vi "Head Co-ordinates 2.vi"(4 "3D Convention":T2(ring), 5 "3D Type and Co-ordinate System":T1(ring), 6 "Sample Rate":dbl format="%.2f", 7 "Array":dbl[][](array[numeric]) format="%.2f") -> (2 "Channel List":string[](array[string]), 3 "3D Output":dbl[][](array[numeric]) format="%.2f")   [LabVIEW 2013]
uses:
  <vilib>/Analysis/baseanly.llb/Real A x B.vi
  <vilib>/Analysis/baseanly.llb/Real Inverse Matrix.vi
  quaternion/quaternion.lvlib
  fick-matrix/fick-matrix.lvlib
  <vilib>/Analysis/NI_AALBase.lvlib
panel:
  # "Copyright Americo A. Migliaccio (c) 2002 All Rights Reserved by Author"
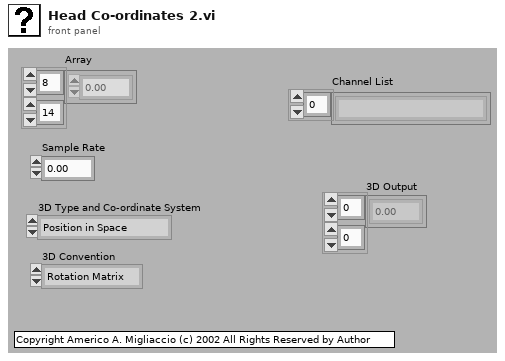
[diagram p1: front panel]
types:
  T1 = enum16{"Position in Space", "Position in Head", "Position in Eye", "Velocity in Space", "Velocity in Head", "Velocity in Eye", "Acceleration in Space", "Acceleration in Head"}
  T2 = enum16{"Rotation Matrix", "Rotation Vectors", "Quaternions", "Fick Angles", "Helmholtz Angles"}
  T3 = typedef "NI_Matrix.lvlib/RealMatrix.ctl" = dbl[][]
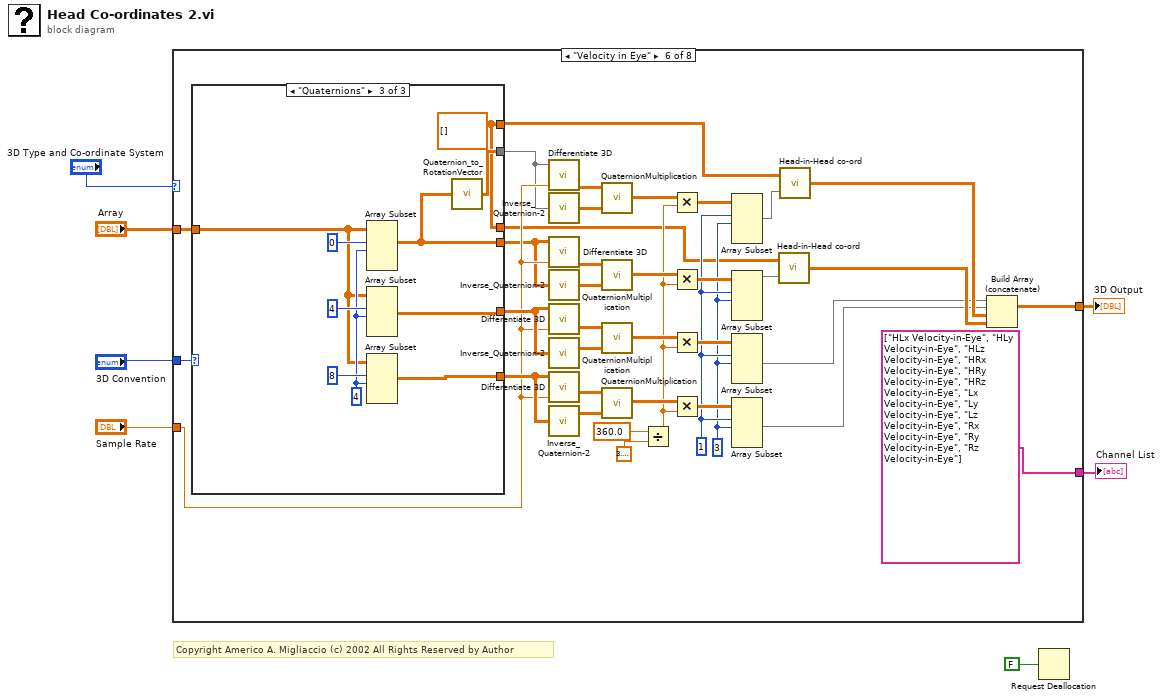
[diagram p0: block diagram]
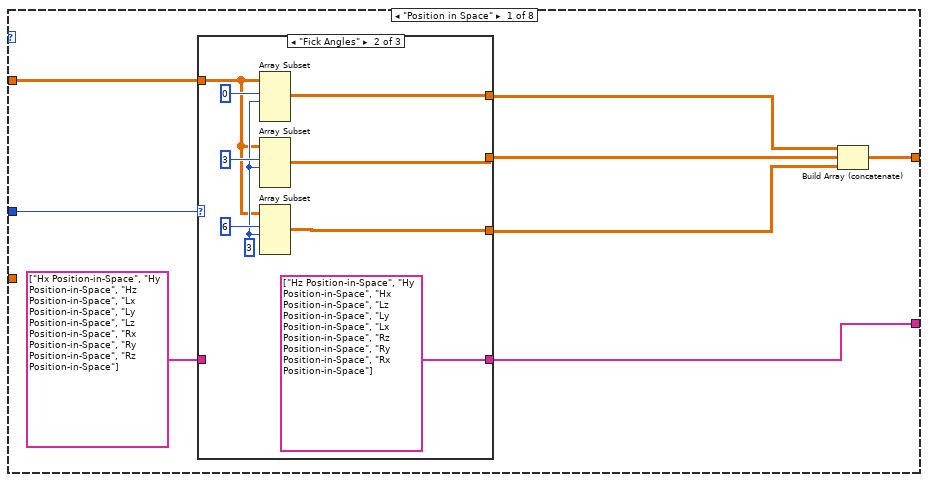
[diagram p2: hidden frame]
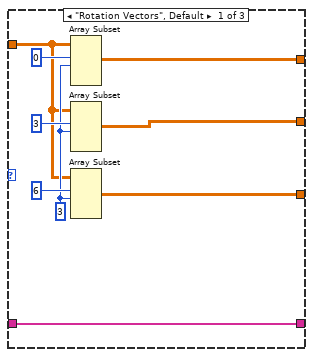
[diagram p3: hidden frame]
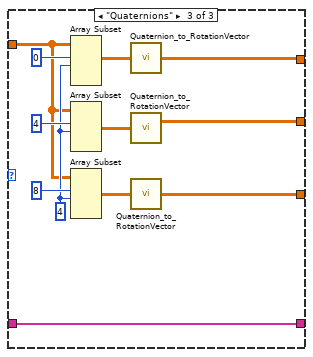
[diagram p4: hidden frame]
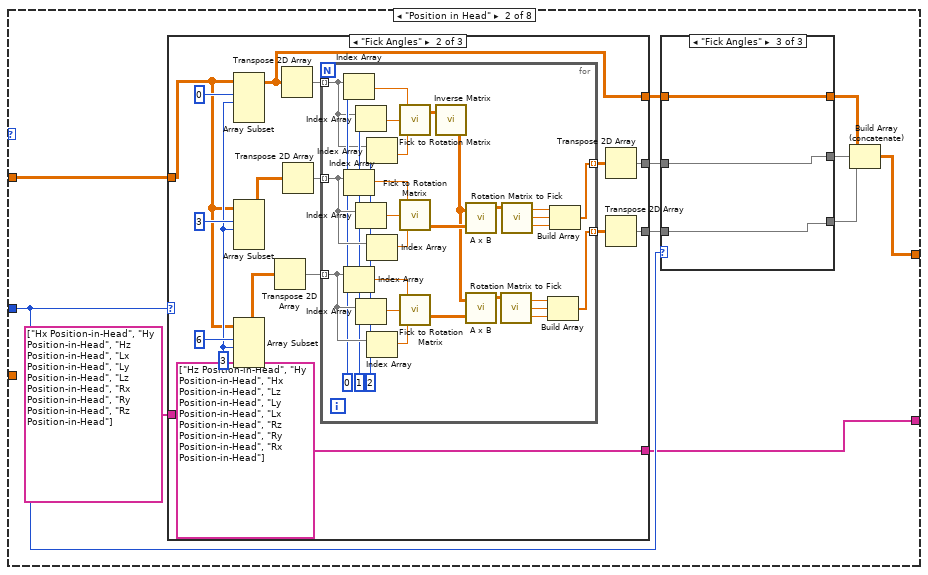
[diagram p5: hidden frame]
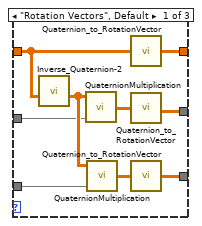
[diagram p6: hidden frame]
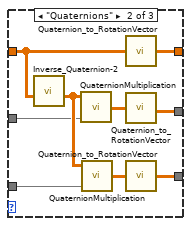
[diagram p7: hidden frame]
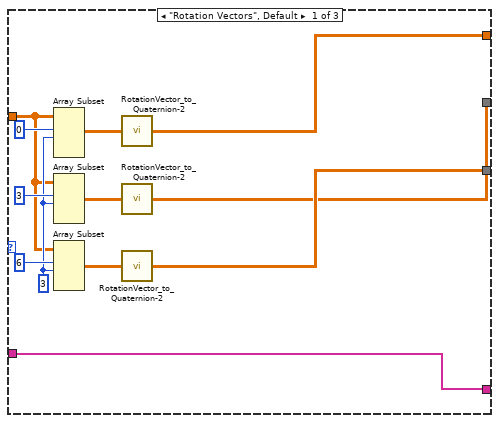
[diagram p8: hidden frame]
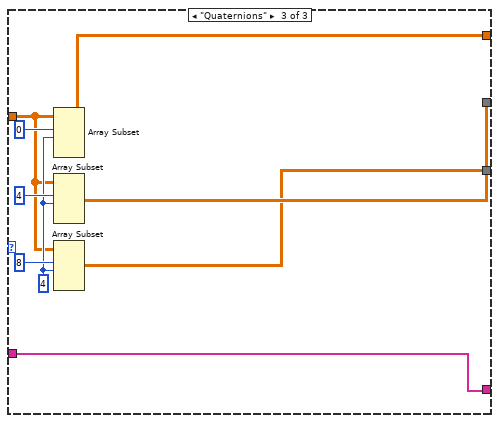
[diagram p9: hidden frame]
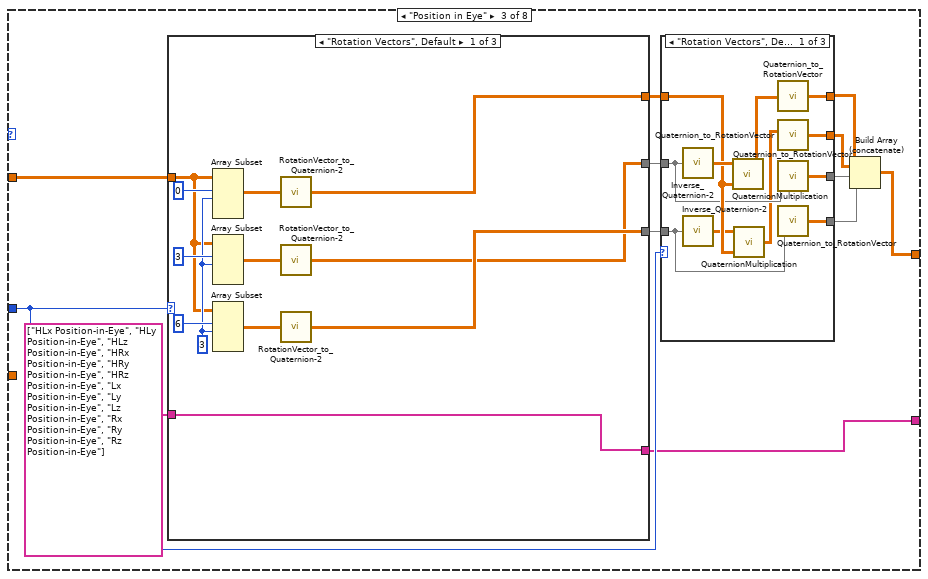
[diagram p10: hidden frame]
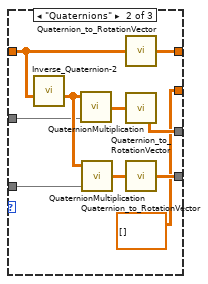
[diagram p11: hidden frame]
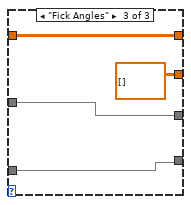
[diagram p12: hidden frame]
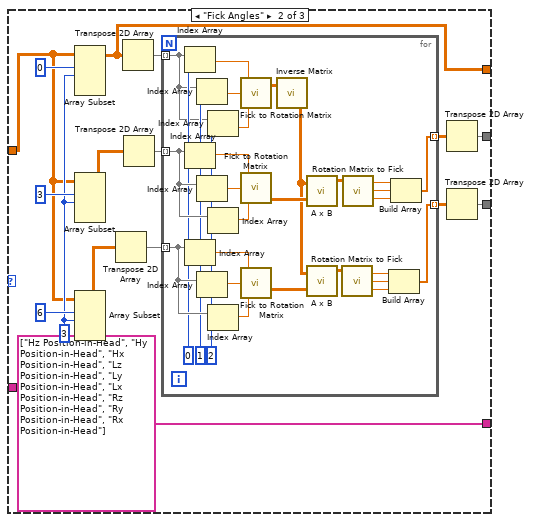
[diagram p13: hidden frame]
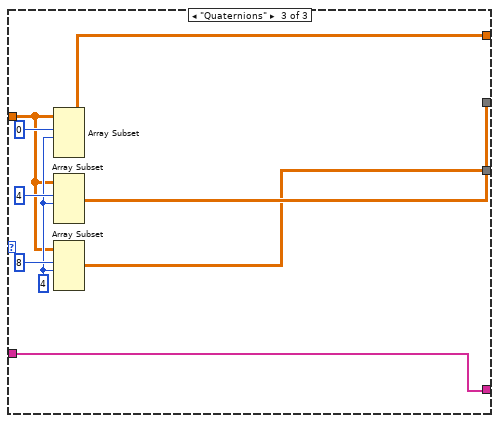
[diagram p14: hidden frame]
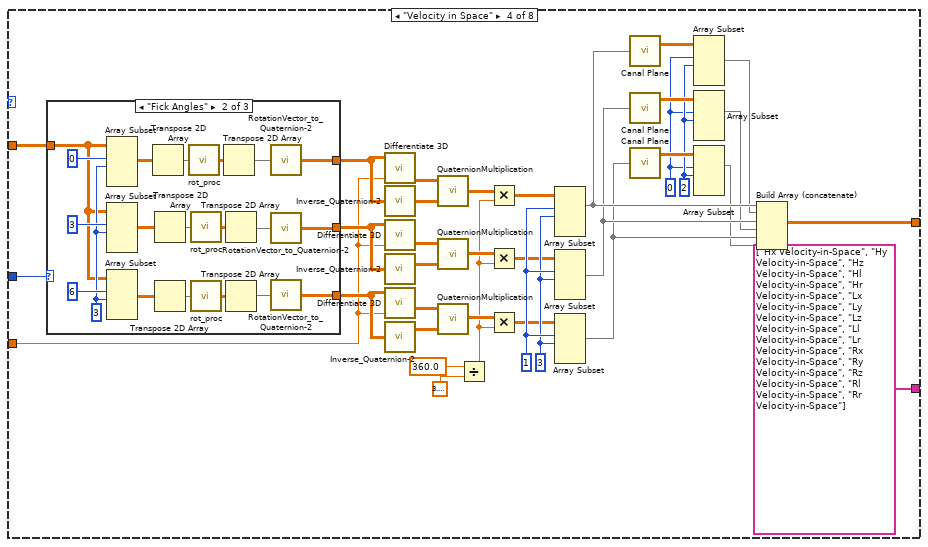
[diagram p15: hidden frame]
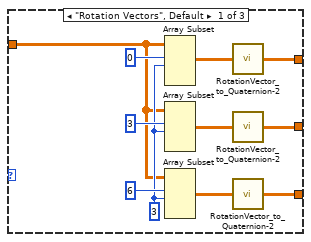
[diagram p16: hidden frame]
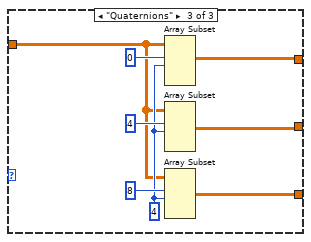
[diagram p17: hidden frame]
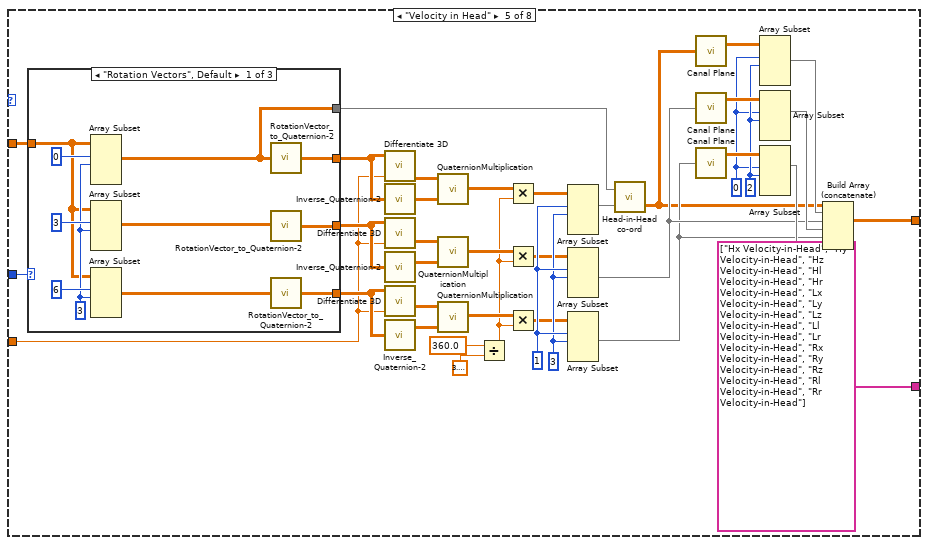
[diagram p18: hidden frame]
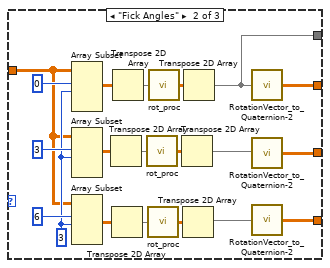
[diagram p19: hidden frame]
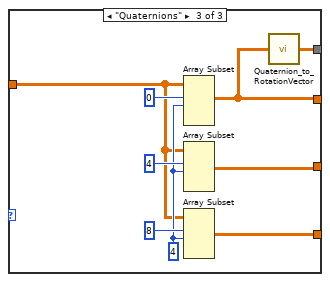
[diagram p20: hidden frame]
diagram:
  # "Copyright Americo A. Migliaccio (c) 2002 All Rights Reserved by Author"
  n1 = case shown="\"Velocity in Eye\"" "3D Type and Co-ordinate System" {
    tunnel: [w10 w50 w150 w263 w327 w420 w484 w498] -> w2
    tunnel: "Array" -> [w15 w48 w148 w282 w359 w437 w496 w510]
    tunnel: "3D Convention" -> [w14 w49 w149 w281 w358 w436 _ _]
    tunnel: "Sample Rate" -> [_ _ _ w264 w338 w408 w488 w502]
    tunnel: [w8 w47 w147 string[] ["Hx Velocity-in-Space", "Hy Velocity-in-Space", "Hz Velocity-in-Space", "Hl Velocity-in-Space", "Hr Velocity-in-Space", "Lx Velocity-in-Space", "Ly Velocity-in-Space", "Lz Velocity-in-Space", "Ll Velocity-in-Space", "Lr Velocity-in-Space", "Rx Velocity-in-Space", "Ry Velocity-in-Space", "Rz Velocity-in-Space", "Rl Velocity-in-Space", "Rr Velocity-in-Space"] ("Channel List") string[] ["Hx Velocity-in-Head", "Hy Velocity-in-Head", "Hz Velocity-in-Head", "Hl Velocity-in-Head", "Hr Velocity-in-Head", "Lx Velocity-in-Head", "Ly Velocity-in-Head", "Lz Velocity-in-Head", "Ll Velocity-in-Head", "Lr Velocity-in-Head", "Rx Velocity-in-Head", "Ry Velocity-in-Head", "Rz Velocity-in-Head", "Rl Velocity-in-Head", "Rr Velocity-in-Head"] ("Channel List") string[] ["HLx Velocity-in-Eye", "HLy Velocity-in-Eye", "HLz Velocity-in-Eye", "HRx Velocity-in-Eye", "HRy Velocity-in-Eye", "HRz Velocity-in-Eye", "Lx Velocity-in-Eye", "Ly Velocity-in-Eye", "Lz Velocity-in-Eye", "Rx Velocity-in-Eye", "Ry Velocity-in-Eye", "Rz Velocity-in-Eye"] ("Channel List") string[] ["Hx Acceleration-in-Space", "Hy Acceleration-in-Space", "Hz Acceleration-in-Space", "Hl Acceleration-in-Space", "Hr Acceleration-in-Space", "Lx Acceleration-in-Space", "Ly Acceleration-in-Space", "Lz Acceleration-in-Space", "Ll Acceleration-in-Space", "Lr Acceleration-in-Space", "Rx Acceleration-in-Space", "Ry Acceleration-in-Space", "Rz Acceleration-in-Space", "Rl Acceleration-in-Space", "Rr Acceleration-in-Space"] ("Channel List") string[] ["Hx Acceleration-in-Head", "Hy Acceleration-in-Head", "Hz Acceleration-in-Head", "Hl Acceleration-in-Head", "Hr Acceleration-in-Head", "Lx Acceleration-in-Head", "Ly Acceleration-in-Head", "Lz Acceleration-in-Head", "Ll Acceleration-in-Head", "Lr Acceleration-in-Head", "Rx Acceleration-in-Head", "Ry Acceleration-in-Head", "Rz Acceleration-in-Head", "Rl Acceleration-in-Head", "Rr Acceleration-in-Head"] ("Channel List")] -> w3
    frame "Position in Space" {
      n2 = case shown="\"Fick Angles\"" w14 {
        tunnel: w15 -> [w20 w29 w41]
        tunnel: [w19 w26 w35] -> w13
        tunnel: [w18 w27 w36] -> w11
        tunnel: [w17 w28 w37] -> w12
        tunnel: string[] ["Hx Position-in-Space", "Hy Position-in-Space", "Hz Position-in-Space", "Lx Position-in-Space", "Ly Position-in-Space", "Lz Position-in-Space", "Rx Position-in-Space", "Ry Position-in-Space", "Rz Position-in-Space"] ("Channel List") -> [w16 _ w34]
        tunnel: [w16 string[] ["Hz Position-in-Space", "Hy Position-in-Space", "Hx Position-in-Space", "Lz Position-in-Space", "Ly Position-in-Space", "Lx Position-in-Space", "Rz Position-in-Space", "Ry Position-in-Space", "Rx Position-in-Space"] ("Channel List") w34] -> w8
        frame "Rotation Vectors", Default {
          w21 = 3 ("Array Length")
          n3 = Array Subset(array=w20, index (row)=0 ("Array Index"), length (row)=w21) -> (w19:dbl[][])  [unwired: 2 in]
          n4 = Array Subset(array=w20, index (row)=3 ("Array Index"), length (row)=w21) -> (w18:dbl[][])  [unwired: 2 in]
          n5 = Array Subset(array=w20, index (row)=6 ("Array Index"), length (row)=w21) -> (w17:dbl[][])  [unwired: 2 in]
        }
        frame "Fick Angles" {
          w30 = 3 ("Array Length")
          n6 = Array Subset(array=w29, index (row)=0 ("Array Index"), length (row)=w30) -> (w26:dbl[][])  [unwired: 2 in]
          n7 = Array Subset(array=w29, index (row)=3 ("Array Index"), length (row)=w30) -> (w27:dbl[][])  [unwired: 2 in]
          n8 = Array Subset(array=w29, index (row)=6 ("Array Index"), length (row)=w30) -> (w28:dbl[][])  [unwired: 2 in]
        }
        frame "Quaternions" {
          w42 = 4 ("Array Length")
          n9 = Array Subset(array=w41, index (row)=0 ("Array Index"), length (row)=w42) -> (w40:dbl[][])  [unwired: 2 in]
          n10 = Array Subset(array=w41, index (row)=4 ("Array Index"), length (row)=w42) -> (w39:dbl[][])  [unwired: 2 in]
          n11 = Array Subset(array=w41, index (row)=8 ("Array Index"), length (row)=w42) -> (w38:dbl[][])  [unwired: 2 in]
          n12 = call "Quaternion_to_RotationVector.vi"("quaternions"=w40) -> ("rotation vectors"=w35:dbl[][])  [unwired: 4 in]
          n13 = call "Quaternion_to_RotationVector.vi"("quaternions"=w39) -> ("rotation vectors"=w36:dbl[][])  [unwired: 4 in]
          n14 = call "Quaternion_to_RotationVector.vi"("quaternions"=w38) -> ("rotation vectors"=w37:dbl[][])  [unwired: 4 in]
        }
      }
      n15 = Build Array (concatenate)(w13, w11, w12) -> (w10:dbl[][])
    }
    frame "Position in Head" {
      n16 = case shown="\"Fick Angles\"" w49 {
        tunnel: w48 -> [w85 w101 w139]
        tunnel: [w79 w91 w138] -> w56
        tunnel: [w80 w93 w137] -> w55
        tunnel: [w81 w92 w136] -> w54
        tunnel: [w78 string[] ["Hz Position-in-Head", "Hy Position-in-Head", "Hx Position-in-Head", "Lz Position-in-Head", "Ly Position-in-Head", "Lx Position-in-Head", "Rz Position-in-Head", "Ry Position-in-Head", "Rx Position-in-Head"] ("Channel List") w135] -> w47
        tunnel: string[] ["Hx Position-in-Head", "Hy Position-in-Head", "Hz Position-in-Head", "Lx Position-in-Head", "Ly Position-in-Head", "Lz Position-in-Head", "Rx Position-in-Head", "Ry Position-in-Head", "Rz Position-in-Head"] ("Channel List") -> [w78 _ w135]
        frame "Rotation Vectors", Default {
          w86 = 3 ("Array Length")
          n17 = Array Subset(array=w85, index (row)=0 ("Array Index"), length (row)=w86) -> (w84:dbl[][])  [unwired: 2 in]
          n18 = Array Subset(array=w85, index (row)=3 ("Array Index"), length (row)=w86) -> (w83:dbl[][])  [unwired: 2 in]
          n19 = Array Subset(array=w85, index (row)=6 ("Array Index"), length (row)=w86) -> (w82:dbl[][])  [unwired: 2 in]
          n20 = call "RotationVector_to_Quaternion-2.vi"("rotation vectors"=w84) -> ("quaternions"=w79:dbl[][])  [unwired: 4 in]
          n21 = call "RotationVector_to_Quaternion-2.vi"("rotation vectors"=w83) -> ("quaternions"=w80:dbl[][])  [unwired: 4 in]
          n22 = call "RotationVector_to_Quaternion-2.vi"("rotation vectors"=w82) -> ("quaternions"=w81:dbl[][])  [unwired: 4 in]
        }
        frame "Fick Angles" {
          w102 = 3 ("Array Length")
          n23 = Array Subset(array=w101, index (row)=0 ("Array Index"), length (row)=w102) -> (w91:dbl[][])  [unwired: 2 in]
          n24 = Array Subset(array=w101, index (row)=3 ("Array Index"), length (row)=w102) -> (w100:dbl[][])  [unwired: 2 in]
          n25 = Array Subset(array=w101, index (row)=6 ("Array Index"), length (row)=w102) -> (w99:dbl[][])  [unwired: 2 in]
          n26 = Transpose 2D Array(2D array=w99) -> (transposed array=w98:dbl[][])
          n27 = Transpose 2D Array(2D array=w91) -> (transposed array=w96:dbl[][])
          n28 = Transpose 2D Array(2D array=w100) -> (transposed array=w97:dbl[][])
          n29 = for {
            tunnel: w96 -> [w110] mode=indexing
            tunnel: w97 -> [w134] mode=indexing
            tunnel: w98 -> [w133] mode=indexing
            tunnel: [w116] -> w95 mode=indexing
            tunnel: [w114] -> w94 mode=indexing
            w130 = 2 ("Array Index")
            w131 = 1 ("Array Index")
            w132 = 0 ("Array Index")
            n30 = Index Array(array=w110, index=w132) -> (element=w113:dbl)
            n31 = Index Array(array=w134, index=w132) -> (element=w127:dbl)
            n32 = Index Array(array=w133, index=w132) -> (element=w124:dbl)
            n33 = Index Array(array=w110, index=w131) -> (element=w112:dbl)
            n34 = Index Array(array=w134, index=w131) -> (element=w128:dbl)
            n35 = Index Array(array=w133, index=w131) -> (element=w126:dbl)
            n36 = Index Array(array=w110, index=w130) -> (element=w111:dbl)
            n37 = Index Array(array=w134, index=w130) -> (element=w129:dbl)
            n38 = Index Array(array=w133, index=w130) -> (element=w125:dbl)
            n39 = call "Fick to Rotation Matrix.vi"("T"=w111, "V"=w112, "H"=w113) -> ("Rotation Matrix"=w123:dbl[][])
            n40 = call "Fick to Rotation Matrix.vi"("T"=w129, "V"=w128, "H"=w127) -> ("Rotation Matrix"=w122:dbl[][])
            n41 = call "Fick to Rotation Matrix.vi"("T"=w125, "V"=w126, "H"=w124) -> ("Rotation Matrix"=w120:dbl[][])
            n42 = call-poly <vilib>:"Inverse Matrix.vi"("Input Matrix"=w123) -> ("Inverse Matrix"=w121:T3)  [unwired: 1 in, 1 out]
            n43 = call-poly <vilib>:"A x B.vi"("B"=w122, "A"=w121) -> ("A x B"=w119:T3)  [unwired: 1 out]
            n44 = call-poly <vilib>:"A x B.vi"("B"=w120, "A"=w121) -> ("A x B"=w118:T3)  [unwired: 1 out]
            n45 = call "Rotation Matrix to Fick.vi"("A"=w118) -> ("T"=w106:dbl, "V"=w115:dbl, "H"=w107:dbl)  [unwired: 2 in]
            n46 = call "Rotation Matrix to Fick.vi"("A"=w119) -> ("T"=w109:dbl, "V"=w117:dbl, "H"=w108:dbl)  [unwired: 2 in]
            n47 = Build Array(w107, w115, w106) -> (w114:dbl[])
            n48 = Build Array(w108, w117, w109) -> (w116:dbl[])
          }
          n49 = Transpose 2D Array(2D array=w95) -> (transposed array=w93:dbl[][])
          n50 = Transpose 2D Array(2D array=w94) -> (transposed array=w92:dbl[][])
        }
        frame "Quaternions" {
          w140 = 4 ("Array Length")
          n51 = Array Subset(array=w139, index (row)=0 ("Array Index"), length (row)=w140) -> (w138:dbl[][])  [unwired: 2 in]
          n52 = Array Subset(array=w139, index (row)=4 ("Array Index"), length (row)=w140) -> (w137:dbl[][])  [unwired: 2 in]
          n53 = Array Subset(array=w139, index (row)=8 ("Array Index"), length (row)=w140) -> (w136:dbl[][])  [unwired: 2 in]
        }
      }
      n54 = case shown="\"Fick Angles\"" w49 {
        tunnel: w56 -> [w62 w71 w75]
        tunnel: w55 -> [w61 w70 w76]
        tunnel: w54 -> [w60 w69 w77]
        tunnel: [w59 w68 w76] -> w53
        tunnel: [w58 w67 w75] -> w52
        tunnel: [w57 w66 w77] -> w51
        frame "Rotation Vectors", Default {
          n55 = call "Inverse_Quaternion-2.vi"("quaternions"=w62) -> ("inverse quaternions"=w64:dbl[][])  [unwired: 4 in]
          n56 = call "QuaternionMultiplication.vi"("quaternions B"=w61, "quaternions A"=w64) -> ("quaternions A x B"=w63:dbl[][])  [unwired: 3 in]
          n57 = call "QuaternionMultiplication.vi"("quaternions B"=w60, "quaternions A"=w64) -> ("quaternions A x B"=w65:dbl[][])  [unwired: 3 in]
          n58 = call "Quaternion_to_RotationVector.vi"("quaternions"=w62) -> ("rotation vectors"=w58:dbl[][])  [unwired: 4 in]
          n59 = call "Quaternion_to_RotationVector.vi"("quaternions"=w63) -> ("rotation vectors"=w59:dbl[][])  [unwired: 4 in]
          n60 = call "Quaternion_to_RotationVector.vi"("quaternions"=w65) -> ("rotation vectors"=w57:dbl[][])  [unwired: 4 in]
        }
        frame "Quaternions" {
          n61 = call "Inverse_Quaternion-2.vi"("quaternions"=w71) -> ("inverse quaternions"=w73:dbl[][])  [unwired: 4 in]
          n62 = call "QuaternionMultiplication.vi"("quaternions B"=w70, "quaternions A"=w73) -> ("quaternions A x B"=w72:dbl[][])  [unwired: 3 in]
          n63 = call "QuaternionMultiplication.vi"("quaternions B"=w69, "quaternions A"=w73) -> ("quaternions A x B"=w74:dbl[][])  [unwired: 3 in]
          n64 = call "Quaternion_to_RotationVector.vi"("quaternions"=w71) -> ("rotation vectors"=w67:dbl[][])  [unwired: 4 in]
          n65 = call "Quaternion_to_RotationVector.vi"("quaternions"=w72) -> ("rotation vectors"=w68:dbl[][])  [unwired: 4 in]
          n66 = call "Quaternion_to_RotationVector.vi"("quaternions"=w74) -> ("rotation vectors"=w66:dbl[][])  [unwired: 4 in]
        }
        frame "Fick Angles" {
        }
      }
      n67 = Build Array (concatenate)(w52, w53, w51) -> (w50:dbl[][])
    }
    frame "Position in Eye" {
      n68 = case shown="\"Rotation Vectors\", Default" w149 {
        tunnel: w148 -> [w188 w204 w242]
        tunnel: [w182 w194 w241] -> w155
        tunnel: [w183 w196 w240] -> w154
        tunnel: [w184 w195 w239] -> w153
        tunnel: [w181 string[] ["Hz Position-in-Head", "Hy Position-in-Head", "Hx Position-in-Head", "Lz Position-in-Head", "Ly Position-in-Head", "Lx Position-in-Head", "Rz Position-in-Head", "Ry Position-in-Head", "Rx Position-in-Head"] ("Channel List") w238] -> w147
        tunnel: string[] ["HLx Position-in-Eye", "HLy Position-in-Eye", "HLz Position-in-Eye", "HRx Position-in-Eye", "HRy Position-in-Eye", "HRz Position-in-Eye", "Lx Position-in-Eye", "Ly Position-in-Eye", "Lz Position-in-Eye", "Rx Position-in-Eye", "Ry Position-in-Eye", "Rz Position-in-Eye"] ("Channel List") -> [w181 _ w238]
        frame "Rotation Vectors", Default {
          w189 = 3 ("Array Length")
          n69 = Array Subset(array=w188, index (row)=0 ("Array Index"), length (row)=w189) -> (w187:dbl[][])  [unwired: 2 in]
          n70 = Array Subset(array=w188, index (row)=3 ("Array Index"), length (row)=w189) -> (w186:dbl[][])  [unwired: 2 in]
          n71 = Array Subset(array=w188, index (row)=6 ("Array Index"), length (row)=w189) -> (w185:dbl[][])  [unwired: 2 in]
          n72 = call "RotationVector_to_Quaternion-2.vi"("rotation vectors"=w187) -> ("quaternions"=w182:dbl[][])  [unwired: 4 in]
          n73 = call "RotationVector_to_Quaternion-2.vi"("rotation vectors"=w186) -> ("quaternions"=w183:dbl[][])  [unwired: 4 in]
          n74 = call "RotationVector_to_Quaternion-2.vi"("rotation vectors"=w185) -> ("quaternions"=w184:dbl[][])  [unwired: 4 in]
        }
        frame "Fick Angles" {
          w205 = 3 ("Array Length")
          n75 = Array Subset(array=w204, index (row)=0 ("Array Index"), length (row)=w205) -> (w194:dbl[][])  [unwired: 2 in]
          n76 = Array Subset(array=w204, index (row)=3 ("Array Index"), length (row)=w205) -> (w203:dbl[][])  [unwired: 2 in]
          n77 = Array Subset(array=w204, index (row)=6 ("Array Index"), length (row)=w205) -> (w202:dbl[][])  [unwired: 2 in]
          n78 = Transpose 2D Array(2D array=w202) -> (transposed array=w201:dbl[][])
          n79 = Transpose 2D Array(2D array=w194) -> (transposed array=w199:dbl[][])
          n80 = Transpose 2D Array(2D array=w203) -> (transposed array=w200:dbl[][])
          n81 = for {
            tunnel: w199 -> [w213] mode=indexing
            tunnel: w200 -> [w237] mode=indexing
            tunnel: w201 -> [w236] mode=indexing
            tunnel: [w219] -> w198 mode=indexing
            tunnel: [w217] -> w197 mode=indexing
            w233 = 2 ("Array Index")
            w234 = 1 ("Array Index")
            w235 = 0 ("Array Index")
            n82 = Index Array(array=w213, index=w235) -> (element=w216:dbl)
            n83 = Index Array(array=w237, index=w235) -> (element=w230:dbl)
            n84 = Index Array(array=w236, index=w235) -> (element=w227:dbl)
            n85 = Index Array(array=w213, index=w234) -> (element=w215:dbl)
            n86 = Index Array(array=w237, index=w234) -> (element=w231:dbl)
            n87 = Index Array(array=w236, index=w234) -> (element=w229:dbl)
            n88 = Index Array(array=w213, index=w233) -> (element=w214:dbl)
            n89 = Index Array(array=w237, index=w233) -> (element=w232:dbl)
            n90 = Index Array(array=w236, index=w233) -> (element=w228:dbl)
            n91 = call "Fick to Rotation Matrix.vi"("T"=w214, "V"=w215, "H"=w216) -> ("Rotation Matrix"=w226:dbl[][])
            n92 = call "Fick to Rotation Matrix.vi"("T"=w232, "V"=w231, "H"=w230) -> ("Rotation Matrix"=w225:dbl[][])
            n93 = call "Fick to Rotation Matrix.vi"("T"=w228, "V"=w229, "H"=w227) -> ("Rotation Matrix"=w223:dbl[][])
            n94 = call-poly <vilib>:"Inverse Matrix.vi"("Input Matrix"=w226) -> ("Inverse Matrix"=w224:T3)  [unwired: 1 in, 1 out]
            n95 = call-poly <vilib>:"A x B.vi"("B"=w225, "A"=w224) -> ("A x B"=w222:T3)  [unwired: 1 out]
            n96 = call-poly <vilib>:"A x B.vi"("B"=w223, "A"=w224) -> ("A x B"=w221:T3)  [unwired: 1 out]
            n97 = call "Rotation Matrix to Fick.vi"("A"=w221) -> ("T"=w209:dbl, "V"=w218:dbl, "H"=w210:dbl)  [unwired: 2 in]
            n98 = call "Rotation Matrix to Fick.vi"("A"=w222) -> ("T"=w212:dbl, "V"=w220:dbl, "H"=w211:dbl)  [unwired: 2 in]
            n99 = Build Array(w210, w218, w209) -> (w217:dbl[])
            n100 = Build Array(w211, w220, w212) -> (w219:dbl[])
          }
          n101 = Transpose 2D Array(2D array=w198) -> (transposed array=w196:dbl[][])
          n102 = Transpose 2D Array(2D array=w197) -> (transposed array=w195:dbl[][])
        }
        frame "Quaternions" {
          w243 = 4 ("Array Length")
          n103 = Array Subset(array=w242, index (row)=0 ("Array Index"), length (row)=w243) -> (w241:dbl[][])  [unwired: 2 in]
          n104 = Array Subset(array=w242, index (row)=4 ("Array Index"), length (row)=w243) -> (w240:dbl[][])  [unwired: 2 in]
          n105 = Array Subset(array=w242, index (row)=8 ("Array Index"), length (row)=w243) -> (w239:dbl[][])  [unwired: 2 in]
        }
      }
      n106 = case shown="\"Rotation Vectors\", Default" w149 {
        tunnel: w155 -> [w161 w173 w178]
        tunnel: w154 -> [w158 w172 w179]
        tunnel: w153 -> [w159 w171 w180]
        tunnel: [w166 w170 w179] -> w152
        tunnel: [w165 w169 w178] -> w145
        tunnel: [w164 w168 w180] -> w151
        tunnel: [w163 dbl[][] [] ("rotation vectors") dbl[][] [] ("rotation vectors")] -> w144
        frame "Rotation Vectors", Default {
          n107 = call "Inverse_Quaternion-2.vi"("quaternions"=w158) -> ("inverse quaternions"=w162:dbl[][])  [unwired: 4 in]
          n108 = call "Inverse_Quaternion-2.vi"("quaternions"=w159) -> ("inverse quaternions"=w160:dbl[][])  [unwired: 4 in]
          n109 = call "QuaternionMultiplication.vi"("quaternions B"=w161, "quaternions A"=w162) -> ("quaternions A x B"=w157:dbl[][])  [unwired: 3 in]
          n110 = call "QuaternionMultiplication.vi"("quaternions B"=w161, "quaternions A"=w160) -> ("quaternions A x B"=w156:dbl[][])  [unwired: 3 in]
          n111 = call "Quaternion_to_RotationVector.vi"("quaternions"=w157) -> ("rotation vectors"=w165:dbl[][])  [unwired: 4 in]
          n112 = call "Quaternion_to_RotationVector.vi"("quaternions"=w156) -> ("rotation vectors"=w163:dbl[][])  [unwired: 4 in]
          n113 = call "Quaternion_to_RotationVector.vi"("quaternions"=w158) -> ("rotation vectors"=w166:dbl[][])  [unwired: 4 in]
          n114 = call "Quaternion_to_RotationVector.vi"("quaternions"=w159) -> ("rotation vectors"=w164:dbl[][])  [unwired: 4 in]
        }
        frame "Quaternions" {
          n115 = call "Inverse_Quaternion-2.vi"("quaternions"=w173) -> ("inverse quaternions"=w175:dbl[][])  [unwired: 4 in]
          n116 = call "QuaternionMultiplication.vi"("quaternions B"=w172, "quaternions A"=w175) -> ("quaternions A x B"=w174:dbl[][])  [unwired: 3 in]
          n117 = call "QuaternionMultiplication.vi"("quaternions B"=w171, "quaternions A"=w175) -> ("quaternions A x B"=w176:dbl[][])  [unwired: 3 in]
          n118 = call "Quaternion_to_RotationVector.vi"("quaternions"=w173) -> ("rotation vectors"=w169:dbl[][])  [unwired: 4 in]
          n119 = call "Quaternion_to_RotationVector.vi"("quaternions"=w174) -> ("rotation vectors"=w170:dbl[][])  [unwired: 4 in]
          n120 = call "Quaternion_to_RotationVector.vi"("quaternions"=w176) -> ("rotation vectors"=w168:dbl[][])  [unwired: 4 in]
        }
        frame "Fick Angles" {
        }
      }
      n121 = Build Array (concatenate)(w145, w144, w152, w151) -> (w150:dbl[][])
    }
    frame "Velocity in Space" {
      w255 = 2 ("Array Index")
      w254 = 0 ("Array Index")
      w280 = 1 ("Array Index")
      w279 = 3 ("Array Index")
      n122 = case shown="\"Fick Angles\"" w281 {
        tunnel: w282 -> [w289 w309 w317]
        tunnel: [w283 w306 w316] -> w267
        tunnel: [w284 w307 w315] -> w266
        tunnel: [w285 w308 w314] -> w265
        frame "Rotation Vectors", Default {
          w290 = 3 ("Array Length")
          n123 = Array Subset(array=w289, index (row)=0 ("Array Index"), length (row)=w290) -> (w288:dbl[][])  [unwired: 2 in]
          n124 = Array Subset(array=w289, index (row)=3 ("Array Index"), length (row)=w290) -> (w287:dbl[][])  [unwired: 2 in]
          n125 = Array Subset(array=w289, index (row)=6 ("Array Index"), length (row)=w290) -> (w286:dbl[][])  [unwired: 2 in]
          n126 = call "RotationVector_to_Quaternion-2.vi"("rotation vectors"=w288) -> ("quaternions"=w283:dbl[][])  [unwired: 4 in]
          n127 = call "RotationVector_to_Quaternion-2.vi"("rotation vectors"=w287) -> ("quaternions"=w284:dbl[][])  [unwired: 4 in]
          n128 = call "RotationVector_to_Quaternion-2.vi"("rotation vectors"=w286) -> ("quaternions"=w285:dbl[][])  [unwired: 4 in]
        }
        frame "Fick Angles" {
          w310 = 3 ("Array Length")
          n129 = Array Subset(array=w309, index (row)=0 ("Array Index"), length (row)=w310) -> (w298:dbl[][])  [unwired: 2 in]
          n130 = Array Subset(array=w309, index (row)=3 ("Array Index"), length (row)=w310) -> (w294:dbl[][])  [unwired: 2 in]
          n131 = Array Subset(array=w309, index (row)=6 ("Array Index"), length (row)=w310) -> (w303:dbl[][])  [unwired: 2 in]
          n132 = Transpose 2D Array(2D array=w298) -> (transposed array=w299:dbl[][])
          n133 = Transpose 2D Array(2D array=w294) -> (transposed array=w301:dbl[][])
          n134 = Transpose 2D Array(2D array=w303) -> (transposed array=w304:dbl[][])
          n135 = call "rot_proc.vi"("Euler Angles"=w299) -> ("Rotation Vectors"=w300:dbl[][])  [unwired: 17 in, 1 out]
          n136 = call "rot_proc.vi"("Euler Angles"=w301) -> ("Rotation Vectors"=w302:dbl[][])  [unwired: 17 in, 1 out]
          n137 = call "rot_proc.vi"("Euler Angles"=w304) -> ("Rotation Vectors"=w305:dbl[][])  [unwired: 17 in, 1 out]
          n138 = Transpose 2D Array(2D array=w300) -> (transposed array=w297:dbl[][])
          n139 = Transpose 2D Array(2D array=w302) -> (transposed array=w296:dbl[][])
          n140 = Transpose 2D Array(2D array=w305) -> (transposed array=w295:dbl[][])
          n141 = call "RotationVector_to_Quaternion-2.vi"("rotation vectors"=w297) -> ("quaternions"=w306:dbl[][])  [unwired: 4 in]
          n142 = call "RotationVector_to_Quaternion-2.vi"("rotation vectors"=w296) -> ("quaternions"=w307:dbl[][])  [unwired: 4 in]
          n143 = call "RotationVector_to_Quaternion-2.vi"("rotation vectors"=w295) -> ("quaternions"=w308:dbl[][])  [unwired: 4 in]
        }
        frame "Quaternions" {
          w318 = 4 ("Array Length")
          n144 = Array Subset(array=w317, index (row)=0 ("Array Index"), length (row)=w318) -> (w316:dbl[][])  [unwired: 2 in]
          n145 = Array Subset(array=w317, index (row)=4 ("Array Index"), length (row)=w318) -> (w315:dbl[][])  [unwired: 2 in]
          n146 = Array Subset(array=w317, index (row)=8 ("Array Index"), length (row)=w318) -> (w314:dbl[][])  [unwired: 2 in]
        }
      }
      n147 = call "Differentiate 3D.vi"("Sample Rate 4"=w264, "Data (in)"=w267) -> ("Data (differentiated)"=w278:dbl[][])  [unwired: 3 in]
      n148 = call "Inverse_Quaternion-2.vi"("quaternions"=w267) -> ("inverse quaternions"=w268:dbl[][])  [unwired: 4 in]
      n149 = call "Differentiate 3D.vi"("Sample Rate 4"=w264, "Data (in)"=w266) -> ("Data (differentiated)"=w270:dbl[][])  [unwired: 3 in]
      n150 = call "Inverse_Quaternion-2.vi"("quaternions"=w266) -> ("inverse quaternions"=w269:dbl[][])  [unwired: 4 in]
      n151 = call "Differentiate 3D.vi"("Sample Rate 4"=w264, "Data (in)"=w265) -> ("Data (differentiated)"=w271:dbl[][])  [unwired: 3 in]
      n152 = call "Inverse_Quaternion-2.vi"("quaternions"=w265) -> ("inverse quaternions"=w272:dbl[][])  [unwired: 4 in]
      n153 = call "QuaternionMultiplication.vi"("quaternions B"=w268, "quaternions A"=w278) -> ("quaternions A x B"=w262:dbl[][])  [unwired: 3 in]
      n154 = call "QuaternionMultiplication.vi"("quaternions B"=w269, "quaternions A"=w270) -> ("quaternions A x B"=w276:dbl[][])  [unwired: 3 in]
      n155 = call "QuaternionMultiplication.vi"("quaternions B"=w272, "quaternions A"=w271) -> ("quaternions A x B"=w277:dbl[][])  [unwired: 3 in]
      n156 = Divide(x=360.0, y=3.141592653589793) -> (x/y=w275:dbl)
      n157 = Multiply(x=w262, y=w275) -> (x*y=w256:dbl[][])
      n158 = Multiply(x=w276, y=w275) -> (x*y=w257:dbl[][])
      n159 = Multiply(x=w277, y=w275) -> (x*y=w258:dbl[][])
      n160 = Array Subset(array=w256, index (row)=w280, length (row)=w279) -> (w253:dbl[][])  [unwired: 2 in]
      n161 = Array Subset(array=w257, index (row)=w280, length (row)=w279) -> (w252:dbl[][])  [unwired: 2 in]
      n162 = Array Subset(array=w258, index (row)=w280, length (row)=w279) -> (w251:dbl[][])  [unwired: 2 in]
      n163 = call "Canal Plane.vi"("Principal Planes"=w253) -> ("Canal Planes"=w259:dbl[][])
      n164 = call "Canal Plane.vi"("Principal Planes"=w252) -> ("Canal Planes"=w260:dbl[][])
      n165 = call "Canal Plane.vi"("Principal Planes"=w251) -> ("Canal Planes"=w261:dbl[][])
      n166 = Array Subset(array=w259, index (row)=w254, length (row)=w255) -> (w250:dbl[][])  [unwired: 2 in]
      n167 = Array Subset(array=w260, index (row)=w254, length (row)=w255) -> (w249:dbl[][])  [unwired: 2 in]
      n168 = Array Subset(array=w261, index (row)=w254, length (row)=w255) -> (w248:dbl[][])  [unwired: 2 in]
      n169 = Build Array (concatenate)(w253, w250, w252, w249, w251, w248) -> (w263:dbl[][])
    }
    frame "Velocity in Head" {
      w334 = 2 ("Array Index")
      w333 = 0 ("Array Index")
      w357 = 1 ("Array Index")
      w356 = 3 ("Array Index")
      n170 = case shown="\"Rotation Vectors\", Default" w358 {
        tunnel: w359 -> [w366 w386 w395]
        tunnel: [w363 w383 w392] -> w341
        tunnel: [w364 w384 w394] -> w340
        tunnel: [w365 w385 w393] -> w339
        tunnel: [w360 w371 w391] -> w325
        frame "Rotation Vectors", Default {
          w367 = 3 ("Array Length")
          n171 = Array Subset(array=w366, index (row)=0 ("Array Index"), length (row)=w367) -> (w360:dbl[][])  [unwired: 2 in]
          n172 = Array Subset(array=w366, index (row)=3 ("Array Index"), length (row)=w367) -> (w361:dbl[][])  [unwired: 2 in]
          n173 = Array Subset(array=w366, index (row)=6 ("Array Index"), length (row)=w367) -> (w362:dbl[][])  [unwired: 2 in]
          n174 = call "RotationVector_to_Quaternion-2.vi"("rotation vectors"=w360) -> ("quaternions"=w363:dbl[][])  [unwired: 4 in]
          n175 = call "RotationVector_to_Quaternion-2.vi"("rotation vectors"=w361) -> ("quaternions"=w364:dbl[][])  [unwired: 4 in]
          n176 = call "RotationVector_to_Quaternion-2.vi"("rotation vectors"=w362) -> ("quaternions"=w365:dbl[][])  [unwired: 4 in]
        }
        frame "Fick Angles" {
          w387 = 3 ("Array Length")
          n177 = Array Subset(array=w386, index (row)=0 ("Array Index"), length (row)=w387) -> (w380:dbl[][])  [unwired: 2 in]
          n178 = Array Subset(array=w386, index (row)=3 ("Array Index"), length (row)=w387) -> (w377:dbl[][])  [unwired: 2 in]
          n179 = Array Subset(array=w386, index (row)=6 ("Array Index"), length (row)=w387) -> (w374:dbl[][])  [unwired: 2 in]
          n180 = Transpose 2D Array(2D array=w377) -> (transposed array=w379:dbl[][])
          n181 = Transpose 2D Array(2D array=w374) -> (transposed array=w376:dbl[][])
          n182 = Transpose 2D Array(2D array=w380) -> (transposed array=w382:dbl[][])
          n183 = call "rot_proc.vi"("Euler Angles"=w379) -> ("Rotation Vectors"=w378:dbl[][])  [unwired: 17 in, 1 out]
          n184 = call "rot_proc.vi"("Euler Angles"=w376) -> ("Rotation Vectors"=w375:dbl[][])  [unwired: 17 in, 1 out]
          n185 = call "rot_proc.vi"("Euler Angles"=w382) -> ("Rotation Vectors"=w381:dbl[][])  [unwired: 17 in, 1 out]
          n186 = Transpose 2D Array(2D array=w378) -> (transposed array=w372:dbl[][])
          n187 = Transpose 2D Array(2D array=w375) -> (transposed array=w373:dbl[][])
          n188 = Transpose 2D Array(2D array=w381) -> (transposed array=w371:dbl[][])
          n189 = call "RotationVector_to_Quaternion-2.vi"("rotation vectors"=w371) -> ("quaternions"=w383:dbl[][])  [unwired: 4 in]
          n190 = call "RotationVector_to_Quaternion-2.vi"("rotation vectors"=w372) -> ("quaternions"=w384:dbl[][])  [unwired: 4 in]
          n191 = call "RotationVector_to_Quaternion-2.vi"("rotation vectors"=w373) -> ("quaternions"=w385:dbl[][])  [unwired: 4 in]
        }
        frame "Quaternions" {
          w396 = 4 ("Array Length")
          n192 = Array Subset(array=w395, index (row)=0 ("Array Index"), length (row)=w396) -> (w392:dbl[][])  [unwired: 2 in]
          n193 = Array Subset(array=w395, index (row)=4 ("Array Index"), length (row)=w396) -> (w394:dbl[][])  [unwired: 2 in]
          n194 = Array Subset(array=w395, index (row)=8 ("Array Index"), length (row)=w396) -> (w393:dbl[][])  [unwired: 2 in]
          n195 = call "Quaternion_to_RotationVector.vi"("quaternions"=w392) -> ("rotation vectors"=w391:dbl[][])  [unwired: 4 in]
        }
      }
      n196 = call "Differentiate 3D.vi"("Sample Rate 4"=w338, "Data (in)"=w341) -> ("Data (differentiated)"=w352:dbl[][])  [unwired: 3 in]
      n197 = call "Inverse_Quaternion-2.vi"("quaternions"=w341) -> ("inverse quaternions"=w342:dbl[][])  [unwired: 4 in]
      n198 = call "Differentiate 3D.vi"("Sample Rate 4"=w338, "Data (in)"=w340) -> ("Data (differentiated)"=w344:dbl[][])  [unwired: 3 in]
      n199 = call "Inverse_Quaternion-2.vi"("quaternions"=w340) -> ("inverse quaternions"=w343:dbl[][])  [unwired: 4 in]
      n200 = call "Differentiate 3D.vi"("Sample Rate 4"=w338, "Data (in)"=w339) -> ("Data (differentiated)"=w345:dbl[][])  [unwired: 3 in]
      n201 = call "Inverse_Quaternion-2.vi"("quaternions"=w339) -> ("inverse quaternions"=w346:dbl[][])  [unwired: 4 in]
      n202 = call "QuaternionMultiplication.vi"("quaternions B"=w342, "quaternions A"=w352) -> ("quaternions A x B"=w324:dbl[][])  [unwired: 3 in]
      n203 = call "QuaternionMultiplication.vi"("quaternions B"=w343, "quaternions A"=w344) -> ("quaternions A x B"=w350:dbl[][])  [unwired: 3 in]
      n204 = call "QuaternionMultiplication.vi"("quaternions B"=w346, "quaternions A"=w345) -> ("quaternions A x B"=w351:dbl[][])  [unwired: 3 in]
      n205 = Divide(x=360.0, y=3.141592653589793) -> (x/y=w349:dbl)
      n206 = Multiply(x=w324, y=w349) -> (x*y=w353:dbl[][])
      n207 = Multiply(x=w350, y=w349) -> (x*y=w354:dbl[][])
      n208 = Multiply(x=w351, y=w349) -> (x*y=w355:dbl[][])
      n209 = Array Subset(array=w353, index (row)=w357, length (row)=w356) -> (w323:dbl[][])  [unwired: 2 in]
      n210 = Array Subset(array=w354, index (row)=w357, length (row)=w356) -> (w329:dbl[][])  [unwired: 2 in]
      n211 = Array Subset(array=w355, index (row)=w357, length (row)=w356) -> (w328:dbl[][])  [unwired: 2 in]
      n212 = call "Head-in-Head co-ord.vi"("Velocity Vector (in space)"=w323, "Rotation Vector (in space)"=w325) -> ("Velocity Vector (in coordinate frame)"=w322:dbl[][])
      n213 = call "Canal Plane.vi"("Principal Planes"=w322) -> ("Canal Planes"=w335:dbl[][])
      n214 = call "Canal Plane.vi"("Principal Planes"=w329) -> ("Canal Planes"=w336:dbl[][])
      n215 = call "Canal Plane.vi"("Principal Planes"=w328) -> ("Canal Planes"=w337:dbl[][])
      n216 = Array Subset(array=w335, index (row)=w333, length (row)=w334) -> (w332:dbl[][])  [unwired: 2 in]
      n217 = Array Subset(array=w336, index (row)=w333, length (row)=w334) -> (w331:dbl[][])  [unwired: 2 in]
      n218 = Array Subset(array=w337, index (row)=w333, length (row)=w334) -> (w330:dbl[][])  [unwired: 2 in]
      n219 = Build Array (concatenate)(w322, w332, w329, w331, w328, w330) -> (w327:dbl[][])
    }
    frame "Velocity in Eye" {
      w411 = 1 ("Array Index")
      w410 = 3 ("Array Index")
      n220 = case shown="\"Quaternions\"" w436 {
        tunnel: w437 -> [w445 w468 w478]
        tunnel: [w442 w465 w475] -> w402
        tunnel: [w441 w466 w477] -> w422
        tunnel: [w440 w467 w476] -> w421
        tunnel: [w443 w453 w474] -> w403
        tunnel: [w439 w452 w473] -> w401
        tunnel: [w438 w452 w473] -> w400
        frame "Rotation Vectors", Default {
          w444 = 3 ("Array Length")
          n221 = Array Subset(array=w445, index (row)=0 ("Array Index"), length (row)=w444) -> (w447:dbl[][])  [unwired: 2 in]
          n222 = Array Subset(array=w445, index (row)=3 ("Array Index"), length (row)=w444) -> (w448:dbl[][])  [unwired: 2 in]
          n223 = Array Subset(array=w445, index (row)=6 ("Array Index"), length (row)=w444) -> (w439:dbl[][])  [unwired: 2 in]
          n224 = Array Subset(array=w445, index (row)=9 ("Array Index"), length (row)=w444) -> (w438:dbl[][])  [unwired: 2 in]
          n225 = call "RotationVector_to_Quaternion-2.vi"("rotation vectors"=w447) -> ("quaternions"=w441:dbl[][])  [unwired: 4 in]
          n226 = call "RotationVector_to_Quaternion-2.vi"("rotation vectors"=w448) -> ("quaternions"=w440:dbl[][])  [unwired: 4 in]
          n227 = call "RotationVector_to_Quaternion-2.vi"("rotation vectors"=w439) -> ("quaternions"=w443:dbl[][])  [unwired: 4 in]
          n228 = call "RotationVector_to_Quaternion-2.vi"("rotation vectors"=w438) -> ("quaternions"=w442:dbl[][])  [unwired: 4 in]
        }
        frame "Fick Angles" {
          w452 = dbl[][] []
          w469 = 3 ("Array Length")
          n229 = Array Subset(array=w468, index (row)=0 ("Array Index"), length (row)=w469) -> (w462:dbl[][])  [unwired: 2 in]
          n230 = Array Subset(array=w468, index (row)=3 ("Array Index"), length (row)=w469) -> (w459:dbl[][])  [unwired: 2 in]
          n231 = Array Subset(array=w468, index (row)=6 ("Array Index"), length (row)=w469) -> (w456:dbl[][])  [unwired: 2 in]
          n232 = Transpose 2D Array(2D array=w459) -> (transposed array=w461:dbl[][])
          n233 = Transpose 2D Array(2D array=w456) -> (transposed array=w458:dbl[][])
          n234 = Transpose 2D Array(2D array=w462) -> (transposed array=w464:dbl[][])
          n235 = call "rot_proc.vi"("Euler Angles"=w461) -> ("Rotation Vectors"=w460:dbl[][])  [unwired: 17 in, 1 out]
          n236 = call "rot_proc.vi"("Euler Angles"=w458) -> ("Rotation Vectors"=w457:dbl[][])  [unwired: 17 in, 1 out]
          n237 = call "rot_proc.vi"("Euler Angles"=w464) -> ("Rotation Vectors"=w463:dbl[][])  [unwired: 17 in, 1 out]
          n238 = Transpose 2D Array(2D array=w460) -> (transposed array=w454:dbl[][])
          n239 = Transpose 2D Array(2D array=w457) -> (transposed array=w455:dbl[][])
          n240 = Transpose 2D Array(2D array=w463) -> (transposed array=w453:dbl[][])
          n241 = call "RotationVector_to_Quaternion-2.vi"("rotation vectors"=w453) -> ("quaternions"=w465:dbl[][])  [unwired: 4 in]
          n242 = call "RotationVector_to_Quaternion-2.vi"("rotation vectors"=w454) -> ("quaternions"=w466:dbl[][])  [unwired: 4 in]
          n243 = call "RotationVector_to_Quaternion-2.vi"("rotation vectors"=w455) -> ("quaternions"=w467:dbl[][])  [unwired: 4 in]
        }
        frame "Quaternions" {
          w473 = dbl[][] []
          w479 = 4 ("Array Length")
          n244 = Array Subset(array=w478, index (row)=0 ("Array Index"), length (row)=w479) -> (w475:dbl[][])  [unwired: 2 in]
          n245 = Array Subset(array=w478, index (row)=4 ("Array Index"), length (row)=w479) -> (w477:dbl[][])  [unwired: 2 in]
          n246 = Array Subset(array=w478, index (row)=8 ("Array Index"), length (row)=w479) -> (w476:dbl[][])  [unwired: 2 in]
          n247 = call "Quaternion_to_RotationVector.vi"("quaternions"=w475) -> ("rotation vectors"=w474:dbl[][])  [unwired: 4 in]
        }
      }
      n248 = call "Differentiate 3D.vi"("Sample Rate 4"=w408, "Data (in)"=w403) -> ("Data (differentiated)"=w416:dbl[][])  [unwired: 3 in]
      n249 = call "Inverse_Quaternion-2.vi"("quaternions"=w403) -> ("inverse quaternions"=w415:dbl[][])  [unwired: 4 in]
      n250 = call "Differentiate 3D.vi"("Sample Rate 4"=w408, "Data (in)"=w402) -> ("Data (differentiated)"=w432:dbl[][])  [unwired: 3 in]
      n251 = call "Inverse_Quaternion-2.vi"("quaternions"=w402) -> ("inverse quaternions"=w423:dbl[][])  [unwired: 4 in]
      n252 = call "Differentiate 3D.vi"("Sample Rate 4"=w408, "Data (in)"=w422) -> ("Data (differentiated)"=w425:dbl[][])  [unwired: 3 in]
      n253 = call "Inverse_Quaternion-2.vi"("quaternions"=w422) -> ("inverse quaternions"=w424:dbl[][])  [unwired: 4 in]
      n254 = call "Differentiate 3D.vi"("Sample Rate 4"=w408, "Data (in)"=w421) -> ("Data (differentiated)"=w426:dbl[][])  [unwired: 3 in]
      n255 = call "Inverse_Quaternion-2.vi"("quaternions"=w421) -> ("inverse quaternions"=w427:dbl[][])  [unwired: 4 in]
      n256 = call "QuaternionMultiplication.vi"("quaternions B"=w415, "quaternions A"=w416) -> ("quaternions A x B"=w414:dbl[][])  [unwired: 3 in]
      n257 = call "QuaternionMultiplication.vi"("quaternions B"=w423, "quaternions A"=w432) -> ("quaternions A x B"=w418:dbl[][])  [unwired: 3 in]
      n258 = call "QuaternionMultiplication.vi"("quaternions B"=w424, "quaternions A"=w425) -> ("quaternions A x B"=w430:dbl[][])  [unwired: 3 in]
      n259 = call "QuaternionMultiplication.vi"("quaternions B"=w427, "quaternions A"=w426) -> ("quaternions A x B"=w431:dbl[][])  [unwired: 3 in]
      n260 = Divide(x=360.0, y=3.141592653589793) -> (x/y=w413:dbl)
      n261 = Multiply(x=w414, y=w413) -> (x*y=w412:dbl[][])
      n262 = Multiply(x=w418, y=w413) -> (x*y=w433:dbl[][])
      n263 = Multiply(x=w430, y=w413) -> (x*y=w434:dbl[][])
      n264 = Multiply(x=w431, y=w413) -> (x*y=w435:dbl[][])
      n265 = Array Subset(array=w412, index (row)=w411, length (row)=w410) -> (w409:dbl[][])  [unwired: 2 in]
      n266 = Array Subset(array=w433, index (row)=w411, length (row)=w410) -> (w417:dbl[][])  [unwired: 2 in]
      n267 = Array Subset(array=w434, index (row)=w411, length (row)=w410) -> (w405:dbl[][])  [unwired: 2 in]
      n268 = Array Subset(array=w435, index (row)=w411, length (row)=w410) -> (w404:dbl[][])  [unwired: 2 in]
      n269 = call "Head-in-Head co-ord.vi"("Velocity Vector (in space)"=w417, "Rotation Vector (in space)"=w400) -> ("Velocity Vector (in coordinate frame)"=w406:dbl[][])
      n270 = call "Head-in-Head co-ord.vi"("Velocity Vector (in space)"=w409, "Rotation Vector (in space)"=w401) -> ("Velocity Vector (in coordinate frame)"=w407:dbl[][])
      n271 = Build Array (concatenate)(w405, w404, w407, w406) -> (w420:dbl[][])
    }
    frame "Acceleration in Space" {
      w492 = 5 ("Array Length")
      n272 = Array Subset(array=w496, index (row)=0 ("Array Index"), length (row)=w492) -> (w491:dbl[][])  [unwired: 2 in]
      n273 = Array Subset(array=w496, index (row)=5 ("Array Index"), length (row)=w492) -> (w490:dbl[][])  [unwired: 2 in]
      n274 = Array Subset(array=w496, index (row)=10 ("Array Index"), length (row)=w492) -> (w489:dbl[][])  [unwired: 2 in]
      n275 = call "Differentiate 3D.vi"("Sample Rate 4"=w488, "Data (in)"=w491) -> ("Data (differentiated)"=w487:dbl[][])  [unwired: 3 in]
      n276 = call "Differentiate 3D.vi"("Sample Rate 4"=w488, "Data (in)"=w490) -> ("Data (differentiated)"=w486:dbl[][])  [unwired: 3 in]
      n277 = call "Differentiate 3D.vi"("Sample Rate 4"=w488, "Data (in)"=w489) -> ("Data (differentiated)"=w485:dbl[][])  [unwired: 3 in]
      n278 = Build Array (concatenate)(w487, w486, w485) -> (w484:dbl[][])
    }
    frame "Acceleration in Head" {
      w506 = 5 ("Array Length")
      n279 = Array Subset(array=w510, index (row)=0 ("Array Index"), length (row)=w506) -> (w505:dbl[][])  [unwired: 2 in]
      n280 = Array Subset(array=w510, index (row)=5 ("Array Index"), length (row)=w506) -> (w504:dbl[][])  [unwired: 2 in]
      n281 = Array Subset(array=w510, index (row)=10 ("Array Index"), length (row)=w506) -> (w503:dbl[][])  [unwired: 2 in]
      n282 = call "Differentiate 3D.vi"("Sample Rate 4"=w502, "Data (in)"=w505) -> ("Data (differentiated)"=w501:dbl[][])  [unwired: 3 in]
      n283 = call "Differentiate 3D.vi"("Sample Rate 4"=w502, "Data (in)"=w504) -> ("Data (differentiated)"=w499:dbl[][])  [unwired: 3 in]
      n284 = call "Differentiate 3D.vi"("Sample Rate 4"=w502, "Data (in)"=w503) -> ("Data (differentiated)"=w500:dbl[][])  [unwired: 3 in]
      n285 = Build Array (concatenate)(w501, w499, w500) -> (w498:dbl[][])
    }
  }
  "3D Output" <- w2
  "Channel List" <- w3
  n286 = Request Deallocation(FALSE ("flag")) -> ()
